vi "picoscopePythonAnalyisForCharge.vi"(8 "error in (no error)":errorcluster, 11 "PicoscopeV2 in":refnum<class "PicoscopeV2.lvclass">) -> (0 "error out":errorcluster, 3 "PicoscopeV2 out":refnum<class "PicoscopeV2.lvclass">)   [LabVIEW 2020, in "PicoscopeV2.lvclass"]
uses:
  PicoscopeV2.lvclass
  OnOffTypeDef.ctl
  PicoscopeV2.lvclass/PicoscopeV2.ctl
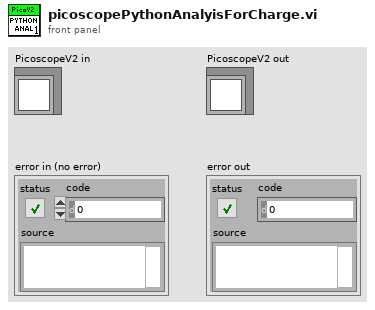
[diagram p1: front panel]
types:
  T1 = typedef "OnOffTypeDef.ctl" = enum16{"off", "on"}
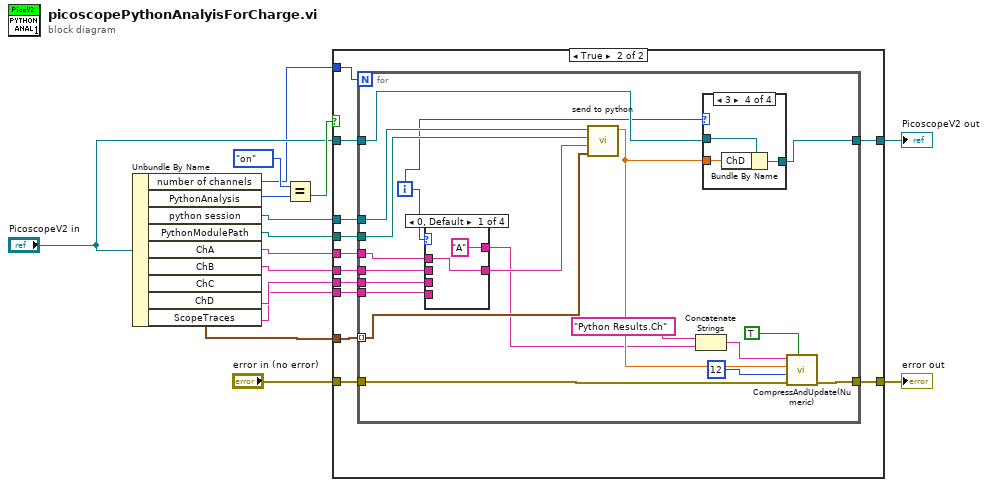
[diagram p0: block diagram]
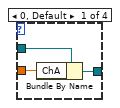
[diagram p3: hidden frame]
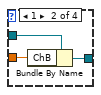
[diagram p4: hidden frame]
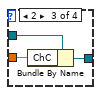
[diagram p5: hidden frame]
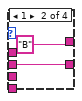
[diagram p6: hidden frame]
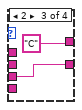
[diagram p7: hidden frame]
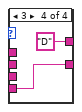
[diagram p8: hidden frame]
diagram:
  n1 = Unbundle By Name("PicoscopeV2 in") -> ("number of channels"=w5:i32, "PythonAnalysis"=w10:T1, "python session"=w13:refnum<k35>, "PythonModulePath"=w14:path, "ChA"=w6:string, "ChB"=w4:string, "ChC"=w2:string, "ChD"=w1:string, "ScopeTraces"=w3:waveform(dbl)[])
  n2 = Equal?(x=OnOffTypeDef."on", y=w10) -> (x = y?=w12:bool)
  n3 = case shown="True" w12 {
    tunnel: w13 -> [_ w29]
    tunnel: w14 -> [_ w28]
    tunnel: w3 -> [_ w27]
    tunnel: "error in (no error)" -> [w16 w24]
    tunnel: [w16 w23] -> w7
    tunnel: "PicoscopeV2 in" -> [w17 w26]
    tunnel: [w17 w25] -> w8
    tunnel: w6 -> [_ w22]
    tunnel: w4 -> [_ w21]
    tunnel: w5 -> [_ w20]
    tunnel: w2 -> [_ w19]
    tunnel: w1 -> [_ w18]
    frame False {
    }
    frame True {
      n4 = for {
        N: w20 -> [_]
        tunnel: w29 -> [w48]
        tunnel: w28 -> [w47]
        tunnel: w27 -> [w33] mode=indexing
        tunnel: w26 -> [w37]
        tunnel: [w35] -> w25
        tunnel: w24 -> [w44]
        tunnel: [w43] -> w23
        tunnel: w22 -> [w40]
        tunnel: w21 -> [w38]
        tunnel: w19 -> [w32]
        tunnel: w18 -> [w31]
        i -> [w34]
        n5 = case shown="0, Default" w34 {
          tunnel: [w62 w64 w66 w68] -> w39
          tunnel: w40 -> [w62 _ _ _]
          tunnel: w38 -> [_ w64 _ _]
          tunnel: w32 -> [_ _ w66 _]
          tunnel: w31 -> [_ _ _ w68]
          tunnel: ["A" "B" "C" "D"] -> w30
          frame 0, Default {
          }
          frame 1 {
          }
          frame 2 {
          }
          frame 3 {
          }
        }
        n6 = call "send to python.vi"("waveform"=w33, "PythonFunctionName"=w39, "PythonModulePath"=w47, "Refnum in"=w48) -> ("result"=w36:dbl)  [unwired: 7 in]
        n7 = Concatenate Strings("Python Results.Ch" ("command or variable name"), w30) -> (w41:string)
        n8 = case shown="3" w34 {
          tunnel: w37 -> [w51 w54 w57 w60]
          tunnel: w36 -> [w50 w53 w56 w59]
          tunnel: [w49 w52 w55 w58] -> w35
          frame 0, Default {
            n9 = Bundle By Name(cluster=w51, "ChA"=w50) -> (w49:refnum<class "PicoscopeV2.lvclass">)
          }
          frame 1 {
            n10 = Bundle By Name(cluster=w54, "ChB"=w53) -> (w52:refnum<class "PicoscopeV2.lvclass">)
          }
          frame 2 {
            n11 = Bundle By Name(cluster=w57, "ChC"=w56) -> (w55:refnum<class "PicoscopeV2.lvclass">)
          }
          frame 3 {
            n12 = Bundle By Name(cluster=w60, "ChD"=w59) -> (w58:refnum<class "PicoscopeV2.lvclass">)
          }
        }
        n13 = call "CompressAndUpdate(Numeric).vi"("force CVT update (false)"=TRUE, "error in"=w44, "precision (6)"=i16 12, "Numeric"=w36, "command or variable name"=w41) -> ("error out"=w43:errorcluster)  [unwired: 6 in]
      }
    }
  }
  "error out" <- w7
  "PicoscopeV2 out" <- w8
